vi "Close.vi"(8 "error in (no error)":errorcluster, 11 "UI Element in":refnum<class "Window.lvclass">) -> (0 "error out":errorcluster)   [LabVIEW 2019, in "Panel.lvlib" / "Window.lvclass"]
doc: "Closes the FP of the window.\n\n----\nPlease see the following web address for additional documentation and tutorial information:\nhttp://www.mooregoodideas.com/mgi-panel-manager/\n\nAuthor: Derek Trepanier\n\nCopyright (c) 2018, Moore Good Ideas, Inc.\n\nAll rights reserved.\n\nRedistribution and use in source and binary forms, with or without modification, are permitted provided that the following conditions are met:\n\n * Redistributions of source code must retain the above copyright notice, this list of conditions and the following disclaimer.\n * Redistributions in binary form must reproduce the above copyright notice, this list of conditions and the following disclaimer in the documentation and/or other materials provided with the distribution.\n * Neither the name of Moore Good Ideas, Inc. nor the names of its contributors may be used to endorse or promote products derived from this software without specific prior written permission.\n\nTHIS SOFTWARE IS PROVIDED BY THE COPYRIGHT HOLDERS AND CONTRIBUTORS \"AS IS\" AND ANY EXPRESS OR IMPLIED WARRANTIES, INCLUDING, BUT NOT LIMITED TO, THE IMPLIED WARRANTIES OF MERCHANTABILITY AND FITNESS FOR A PARTICULAR PURPOSE ARE DISCLAIMED. IN NO EVENT SHALL THE COPYRIGHT OWNER OR CONTRIBUTORS BE LIABLE FOR ANY DIRECT, INDIRECT, INCIDENTAL, SPECIAL, EXEMPLARY, OR CONSEQUENTIAL DAMAGES (INCLUDING, BUT NOT LIMITED TO, PROCUREMENT OF SUBSTITUTE GOODS OR SERVICES; LOSS OF USE, DATA, OR PROFITS; OR BUSINESS INTERRUPTION) HOWEVER CAUSED AND ON ANY THEORY OF LIABILITY, WHETHER IN CONTRACT, STRICT LIABILITY, OR TORT (INCLUDING NEGLIGENCE OR OTHERWISE) ARISING IN ANY WAY OUT OF THE USE OF THIS SOFTWARE, EVEN IF ADVISED OF THE POSSIBILITY OF SUCH DAMAGE."
uses:
  Window.lvclass
  C:/Users/Public/Documents/Development/Drivers/Source/Utilities/Actor Framework Tools/Panel Manager/Panel/Panel/Panel.lvclass
  Panel.lvclass/Panel.ctl
  Window.lvclass/Window.ctl
  Panel.lvclass
  Window Position/Window Position.lvclass
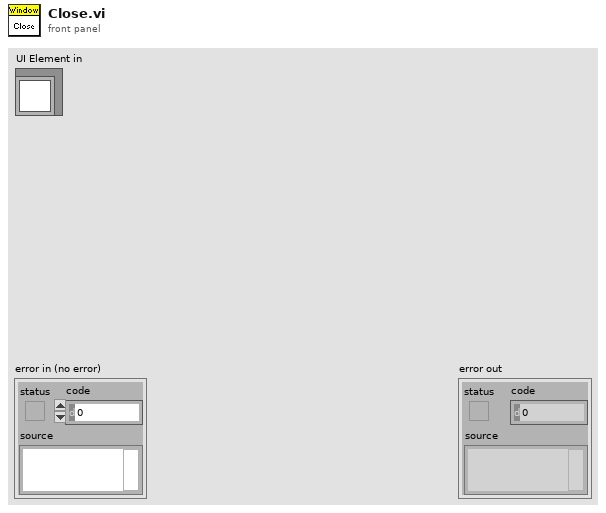
[diagram p1: front panel]
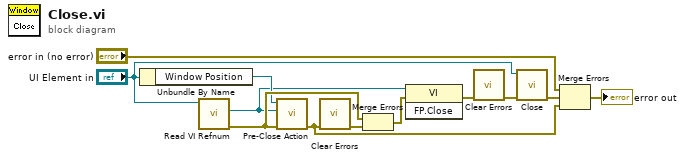
[diagram p0: block diagram]
diagram:
  n1 = Unbundle By Name("UI Element in") -> ("Window Position"=w2:refnum<class "Window Position.lvclass">)
  n2 = call "Read VI Refnum.vi"("Panel in"="UI Element in") -> ("error out"=w7:errorcluster, "VI Refnum"=w1:refnum<vi>)  [unwired: 9 in]
  n3 = call-dynamic "Pre-Close Action.vi"("error in (no error)"=w7, "Panel VI"=w1, "Window Position in"=w2) -> ("error out"=w5:errorcluster)  [unwired: 8 in]
  n4 = call <vilib>:"Clear Errors.vi"("error in (no error)"=w5) -> ("error out"=w4:errorcluster)  [unwired: 5 in, 1 out]
  n5 = Merge Errors(w7, w4) -> (w6:errorcluster)
  n6 = invoke class="VI" method="FP.Close"(reference=w1, error in=w6) -> (error out=w12:errorcluster)  [unwired: 1 in, 2 out]
  n7 = call <vilib>:"Clear Errors.vi"("error in (no error)"=w12) -> ("error out"=w8:errorcluster)  [unwired: 5 in, 1 out]
  n8 = call-parent "Close.vi"("Error In"=w8, "Panel In"="UI Element in") -> ("Error Out"=w9:errorcluster)  [unwired: 9 in]
  n9 = Merge Errors("error in (no error)", w9, w5) -> (→"error out":errorcluster)
